vi "Work.vi"(0 "Action":T5, 6 "Tags":T3, 8 "Init":T4, 9 "State in":T2) -> (11 "State out":T2, 14 "Control":T1={"Skip Next Read"=FALSE, "Skip Write"=FALSE, "Read Timeout"=-1}, 19 "Error":errorcluster)   [LabVIEW 2022 SP3, in "Worker Template.lvlib"]
uses:
  Worker Template.lvlib
  FlexBlocks Support/Worker Action.ctl
  FlexBlocks Support/FlexBlocks Support.lvlib
  Init.ctl
  Tags.ctl
  State.ctl
  FlexBlocks Support/Block IO Control.ctl
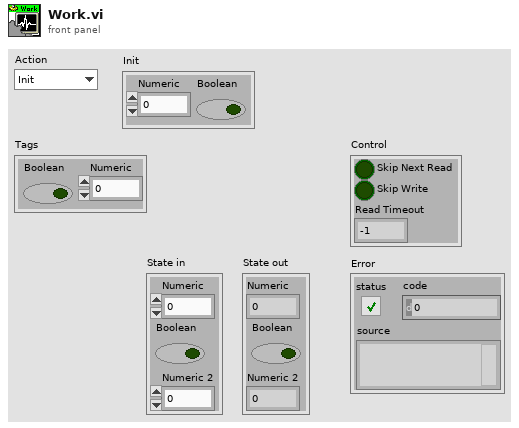
[diagram p1: front panel]
types:
  T1 = typedef "FlexBlocks Support.lvlib/Block IO Control.ctl" = cluster{"Skip Next Read":bool, "Skip Write":bool, "Read Timeout":i32}
  T2 = typedef "Worker Template.lvlib/State.ctl" = cluster{"Numeric":dbl, "Boolean":bool, "Numeric 2":dbl}
  T3 = typedef "Worker Template.lvlib/Tags.ctl" = cluster{"Boolean":bool, "Numeric":dbl}
  T4 = typedef "Worker Template.lvlib/Init.ctl" = cluster{"Numeric":dbl, "Boolean":bool}
  T5 = typedef "FlexBlocks Support.lvlib/Worker Action.ctl" = enum16{"Init", "Start", "Run", "Stop", "Close"}
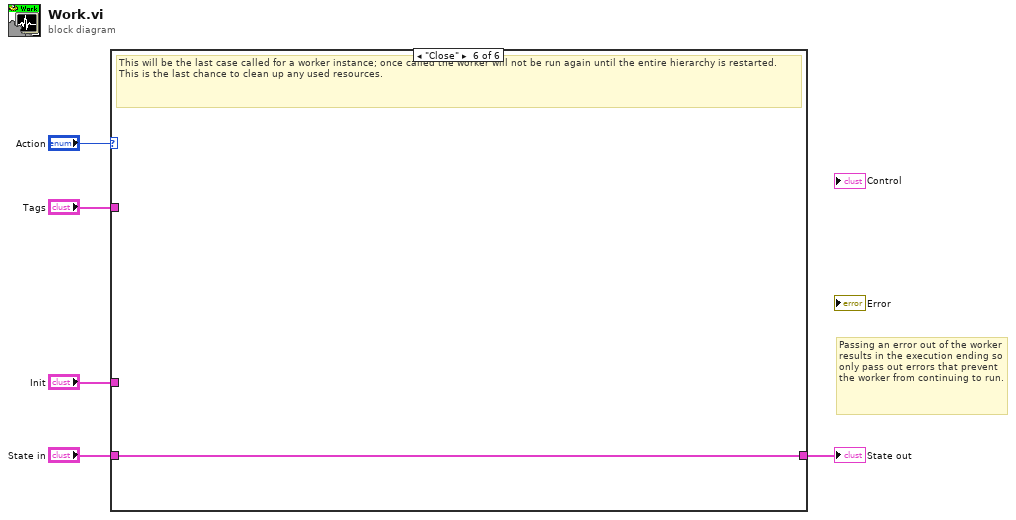
[diagram p0: block diagram]
diagram:
  # "Passing an error out of the worker results in the execution ending so only pass out errors that prevent the worker from continuing to run."
  n1 = case shown="\"Close\"" "Action" {
    tunnel: "State in" -> [w6 w7 w8 w9 w10 w11]
    tunnel: [w6 w7 w8 w9 w10 w11] -> w4
    tunnel: "Init" -> [_ _ _ _ _ _]
    tunnel: "Tags" -> [_ _ _ _ _ _]
    frame Default {
      # "This case is for unused worker actions and should be left empty other than passing the state through."
    }
    frame "Init" {
      # "Called once when the worker is first created so that it can perform initialization logic before starting any work. Note that the worker may not start right away after Init is called so any logic in Init should be done expecting an unknown amount of time to pass before the worker is Started and Run. This usually means not connecting to any devices or beginning any hardware sessions that expect continuous data or will timeout. Such connections can be established in the Start case."
    }
    frame "Start" {
      # "Called immediately before running. This case can be used to open handles to devices and get the worker ready to run."
    }
    frame "Run" {
      # "This is the case where work / processing should be done. All tag input (lossy) and lossless inputs will be up to date when Run is called and any output will be sent along to the next worker or display. Note that this is the only case where outputs are handled and any values output in other cases will be ignored."
    }
    frame "Stop" {
      # "Called when the worker is being put into a paused state but may be started again. This is the case where streaming sessions and device handles that will timeout should be closed."
    }
    frame "Close" {
      # "This will be the last case called for a worker instance; once called the worker will not be run again until the entire hierarchy is restarted. This is the last chance to clean up any used resources."
    }
  }
  "State out" <- w4
